vi "Tektronix 7000 Series Runt Triggered Acquisition Waveform.vi"() -> ()   [LabVIEW 2015]
doc: "This example VI illustrates how to configure an oscilloscope to generate a Runt trigger and acquire a waveform from that trigger."
uses:
  <instrlib>/Tektronix 7000 Series/Public/Configure/Configure Trigger (Runt).vi
  <instrlib>/Tektronix 7000 Series/Public/Data/Read (Single Waveform).vi
  <instrlib>/Tektronix 7000 Series/Tektronix 7000 Series.lvlib
panel:
  in  "Lower Level (0.8V)":dbl=0.8
  in  "Upper Level (1.2V)":dbl=1.2
  in  "Polarity (0:Positive)":u16(ring) items=["Positive", "Negative", "Either"]
  in  "Runt Width (500E-12s)":dbl=5e-10
  out "Waveform Graph":waveform(dbl)(graph)
  in  "Trigger Level (0.0)":dbl
  in  "VISA Resource Name":refnum<visa-resource-name>
  in  "Channel (0: Channel 1)":u16(ring) format="%#_5f" items=["Channel 1", "Channel 2", "Channel 3", "Channel 4", "Math 1", "Math 2", "Math 3", "Math 4", "Reference 1", "Reference 2", "Reference 3", "Reference 4"]
  in  "Vertical Coupling (1: DC)":u16(ring)=1 items=["AC", "DC", "Ground"]
  in  "Timebase (0.005 s)":dbl=0.005
  in  "Vertical Range (10.0 V)":dbl=10.0
  in  "Probe Attenuation (10.0)":dbl=10.0
  # "(c) 2006 - 2016 National Instruments Corporation.  ALL RIGHTS RESERVED."
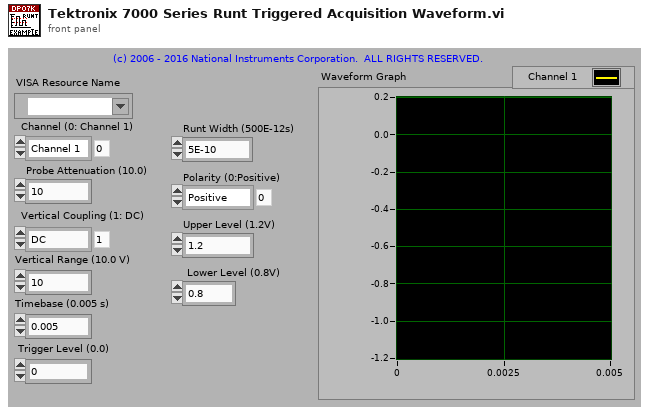
[diagram p1: front panel]
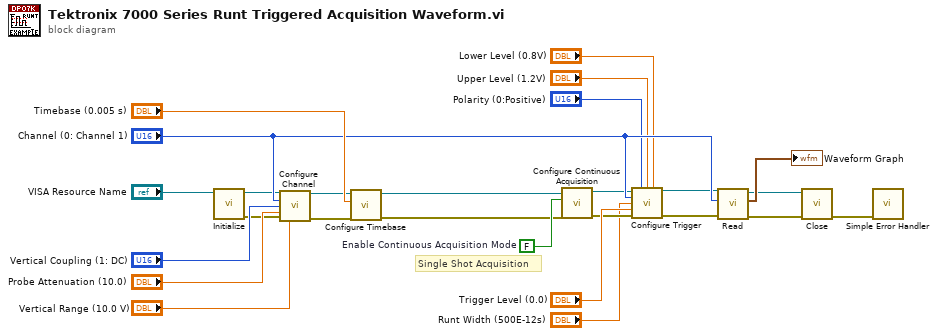
[diagram p0: block diagram]
diagram:
  w12 = FALSE  # Enable Continuous Acquisition Mode
  # "Single Shot Acquisition"
  n1 = call <instrlib>:"Initialize.vi"("VISA resource name"="VISA Resource Name") -> ("error out"=w9:errorcluster, "VISA resource name out"=w8:refnum<visa-resource-name>)  [unwired: 9 in]
  n2 = call <instrlib>:"Configure Channel.vi"("VISA resource name"=w8, "Channel (0: Channel 1)"="Channel (0: Channel 1)", "Vertical Coupling (1: DC)"="Vertical Coupling (1: DC)", "Probe Attenuation (1.0)"="Probe Attenuation (10.0)", "error in (no error)"=w9, "Vertical Range (10.0 V)"="Vertical Range (10.0 V)") -> ("VISA resource name out"=w7:refnum<visa-resource-name>, "error out"=w6:errorcluster)  [unwired: 8 in]
  n3 = call <instrlib>:"Configure Timebase.vi"("error in (no error)"=w6, "Timebase (4 ns)"="Timebase (0.005 s)", "VISA resource name"=w7) -> ("error out"=w11:errorcluster, "VISA resource name out"=w10:refnum<visa-resource-name>)  [unwired: 7 in]
  n4 = call <instrlib>:"Configure Continuous Acquisition.vi"("error in (no error)"=w11, "Enable Continuous Acquisition Mode (True)"=w12, "VISA resource name"=w10) -> ("error out"=w14:errorcluster, "VISA resource name out"=w13:refnum<visa-resource-name>)  [unwired: 7 in]
  n5 = call-poly <instrlib>:"Configure Trigger.vi"("VISA resource name"=w13, "Polarity (0:Positive)"="Polarity (0:Positive)", "Upper Level (1.2V)"="Upper Level (1.2V)", "Lower Level (0.8V)"="Lower Level (0.8V)", "Source (0:Channel1)"="Channel (0: Channel 1)", "Trigger Condition (1: Wider than)"="Runt Width (500E-12s)", "Runt Width (500E-12s)"="Trigger Level (0.0)", "error in (no error)"=w14) -> ("VISA resource name out"=w15:refnum<visa-resource-name>, "error out"=w16:errorcluster)  [unwired: 5 in, 1 out]
  n6 = call-poly <instrlib>:"Read.vi"("error in (no error)"=w16, "Channel (0: Channel 1)"="Channel (0: Channel 1)", "VISA resource name"=w15) -> ("error out"=w19:errorcluster, "Waveform Data"=→"Waveform Graph":waveform(dbl), "VISA resource name out"=w18:refnum<visa-resource-name>)  [unwired: 6 in]
  n7 = call <instrlib>:"Close.vi"("error in (no error)"=w19, "VISA resource name"=w18) -> ("error out"=w17:errorcluster)  [unwired: 9 in]
  n8 = call <vilib>:"Simple Error Handler.vi"("error in (no error)"=w17) -> ()  [unwired: 4 in, 5 out]
